vi "place empty zero value in front of single dig values.vi"(11 "input string value of numeric":string) -> (3 "formated resulting string":string)   [LabVIEW 2010]
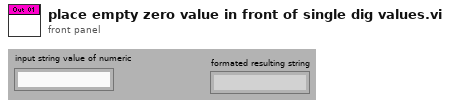
[diagram p1: front panel]
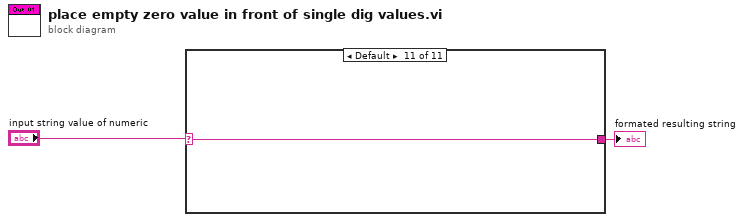
[diagram p0: block diagram]
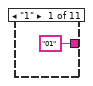
[diagram p2: hidden frame]
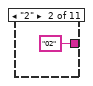
[diagram p3: hidden frame]
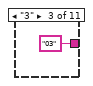
[diagram p4: hidden frame]
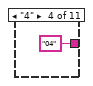
[diagram p5: hidden frame]
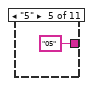
[diagram p6: hidden frame]
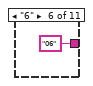
[diagram p7: hidden frame]
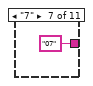
[diagram p8: hidden frame]
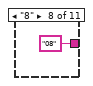
[diagram p9: hidden frame]
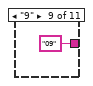
[diagram p10: hidden frame]
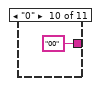
[diagram p11: hidden frame]
diagram:
  n1 = case shown="Default" "input string value of numeric" {
    selector: "input string value of numeric" -> [_ _ _ _ _ _ _ _ _ _ w13]
    tunnel: ["01" "02" "03" "04" "05" "06" "07" "08" "09" "00" w13] -> w1
    frame "1" {
    }
    frame "2" {
    }
    frame "3" {
    }
    frame "4" {
    }
    frame "5" {
    }
    frame "6" {
    }
    frame "7" {
    }
    frame "8" {
    }
    frame "9" {
    }
    frame "0" {
    }
    frame Default {
    }
  }
  "formated resulting string" <- w1
